vi "Pixel count.vi"(11 "Histogram 图标":u32[][](graph)) -> (0 "像素白个数":u32, 3 "像素黑个数":u32)   [LabVIEW 2017]
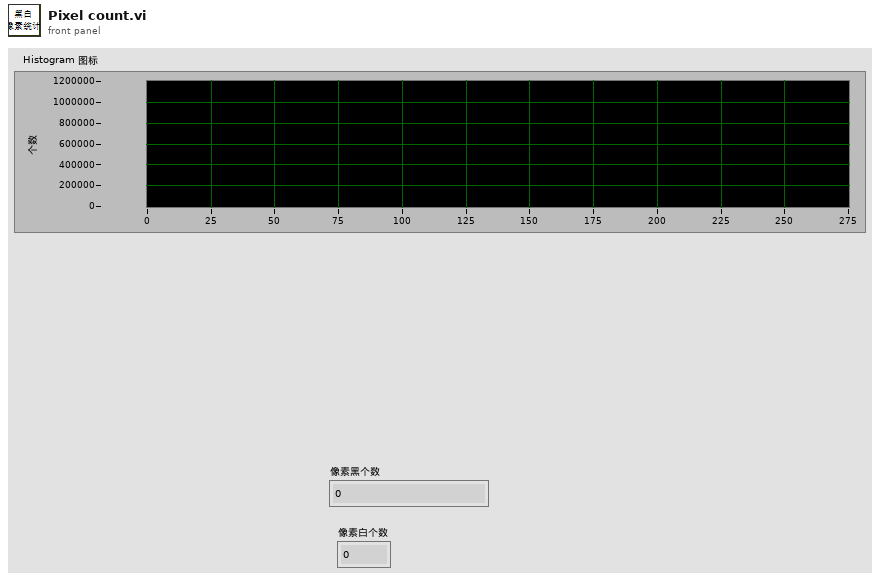
[diagram p1: front panel]
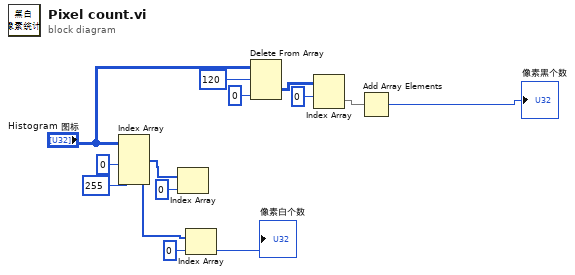
[diagram p0: block diagram]
diagram:
  n1 = Index Array(array="Histogram 图标", index (col) #1=0 ("禁用的索引 (列)"), index (col) #2=255 ("索引 (列)")) -> (element #1=w13:u32[], element #2=w8:u32[])  [unwired: 2 in]
  n2 = Index Array(array=w13, index=0 ("索引")) -> ()  [unwired: 1 out]
  n3 = Index Array(array=w8, index=0 ("索引")) -> (element=→"像素白个数":u32)
  n4 = Delete From Array(array="Histogram 图标", length=120 ("长度"), index (col)=0 ("禁用的索引 (列)")) -> (deleted portion=w4:u32[][])  [unwired: 1 in, 1 out]
  n5 = Index Array(array=w4, index (row)=0 ("索引 (行)")) -> (element=w2:u32[])  [unwired: 1 in]
  n6 = Add Array Elements(numeric array=w2) -> (sum=→"像素黑个数":u32)
